vi "Text0002.vi"   [LabVIEW 2013]
uses:
  <vilib>/Heliosphere Research LLC/Advanced Plotting Toolkit/Advanced Plotting Toolkit.lvlib
types:
  T1 = typedef "Advanced Plotting Toolkit.lvlib/PlotID.ctl" = i32
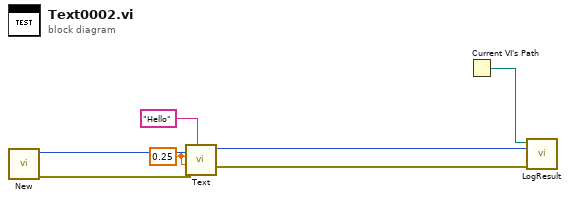
[diagram p0: block diagram]
diagram:
  w6 = 0.25 ("X Position")
  n1 = call <vilib>:"New.vi"() -> ("error out"=w3:errorcluster, "Plot ID"=w4:T1)  [unwired: 10 in]
  n2 = call <vilib>:"Text.vi"("Text"="Hello", "error in (no error)"=w3, "Y Position"=w6, "X Position"=w6, "Plot ID"=w4) -> ("error out"=w1:errorcluster, "Plot ID Out"=w2:T1)  [unwired: 5 in]
  n3 = Current VI's Path() -> (path=w7:path)
  n4 = call "LogResult.vi"("Test Result"=w1, "Test Artifact"=w2, "VI Path"=w7) -> ()  [unwired: 9 in]
